vi "Get SMO HELP.vi"(8 "error in (no error)":errorcluster, 10 "Command":string, 11 "Instrument.Framework-Template in":refnum<class "Instrument.Framework-Template.lvclass">) -> (0 "error out":errorcluster, 2 "output cluster":T1, 3 "Instrument.Framework-Template out":refnum<class "Instrument.Framework-Template.lvclass">)   [LabVIEW 2019, in "Instrument.Framework-Template.lvclass"]
uses:
  Instrument.Framework-Template.lvclass
  Framework/Instrument/Help/typedefs/Help--cluster.ctl
  Typedefs/Instrument.Framework-Template.PublicCommands--Enum.ctl
  Framework/Instrument Types/SCPI/Instrument.SCPI.lvclass
  Framework/Instrument/Help/Help.lvclass
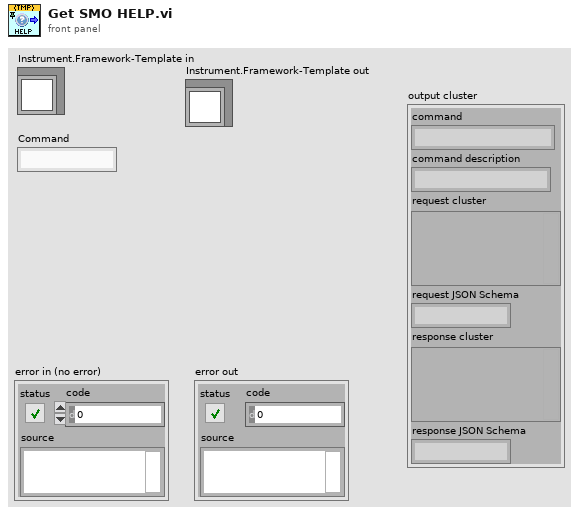
[diagram p1: front panel]
types:
  T1 = typedef "Help.lvclass/Help--cluster.ctl" = cluster{"command":string, "command description":string, "request cluster":variant, "request JSON Schema":string, "response cluster":variant, "response JSON Schema":string}
  T2 = typedef "Instrument.Framework-Template.lvclass/Instrument.Framework-Template.PublicCommands--Enum.ctl" = enum16{"doSomething"}
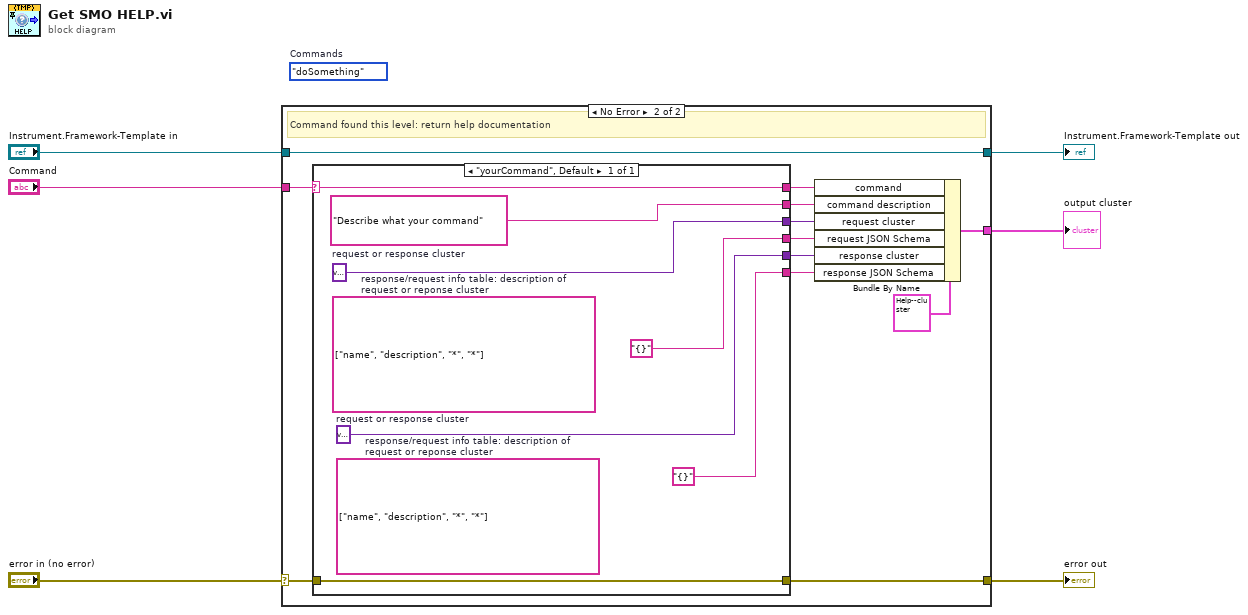
[diagram p0: block diagram]
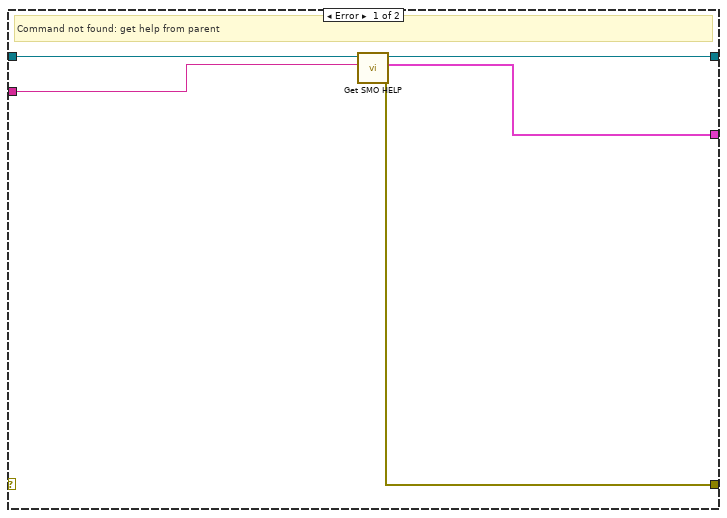
[diagram p2: hidden frame]
diagram:
  (unwired) Instrument.Framework-Template.PublicCommands--Enum."doSomething"  # Commands
  n1 = case shown="No Error" "error in (no error)" {
    selector: "error in (no error)" -> [_ w18]
    tunnel: "Instrument.Framework-Template in" -> [w11 w23]
    tunnel: [w10 w23] -> w5
    tunnel: [w8 w17] -> w6
    tunnel: [w7 w22] -> w4
    tunnel: "Command" -> [w9 w20]
    frame Error {
      # "Command not found: get help from parent"
      n2 = call-parent "Get SMO HELP.vi"("Command"=w9, "Instrument in"=w11) -> ("error out"=w8:errorcluster, "help cluster"=w7:T1, "Instrument out"=w10:refnum<class "Instrument.Framework-Template.lvclass">)  [unwired: 7 in]
    }
    frame No Error {
      # "Command found this level: return help documentation"
      n3 = case shown="\"yourCommand\", Default" w20 {
        selector: w20 -> [w30]
        tunnel: [w30] -> w19
        tunnel: w18 -> [w29]
        tunnel: [w29] -> w17
        tunnel: ["Describe what your command"] -> w16
        tunnel: [w27] -> w15
        tunnel: ["{}"] -> w14
        tunnel: [w26] -> w13
        tunnel: ["{}"] -> w12
        frame "yourCommand", Default {
          w27 = variant  # request or response cluster
          (unwired) string[][] [["name", "description"], ["*", "*"]]  # response/request info table: description of request or reponse cluster
          w26 = variant  # request or response cluster
          (unwired) string[][] [["name", "description"], ["*", "*"]]  # response/request info table: description of request or reponse cluster
        }
      }
      n4 = Bundle By Name(cluster=T1 {"command"="", "command description"="", "request cluster"=variant, "request JSON Schema"="", "response cluster"=variant, "response JSON Schema"=""} ("Help"), "command"=w19, "command description"=w16, "request cluster"=w15, "request JSON Schema"=w14, "response cluster"=w13, "response JSON Schema"=w12) -> (w22:T1)
    }
  }
  "Instrument.Framework-Template out" <- w5
  "output cluster" <- w4
  "error out" <- w6
